vi "mod_Integer Rate Interpolation.vi"(4 "flush buffers? (F)":bool, 6 "reset? (T)":bool=TRUE, 9 "interpolation factor":i32=10, 11 "input[]":cdb[](array[numeric])) -> (3 "output[]":cdb[](array[numeric]), 5 "filter coefficients out[]":dbl[](array[numeric]))   [LabVIEW 2020, in "niAMT.lvlib"]
uses:
  <vilib>/addons/Modulation/niAMT.lvlib
  <vilib>/addons/Modulation/Analog/controls/mod_Integer Interpolator State.ctl
  nilvamt.dll
panel:
  in  "default state":T1
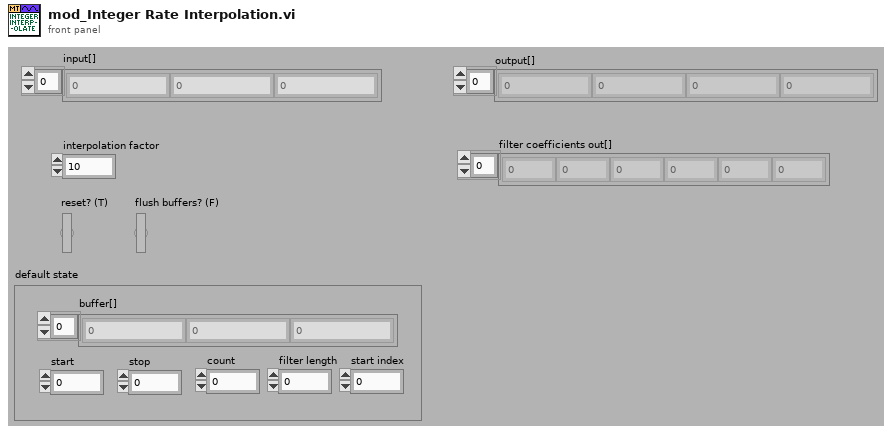
[diagram p1: front panel]
types:
  T1 = typedef "niAMT.lvlib/mod_Integer Interpolator State.ctl" = cluster{"buffer[]":cdb[], "start":i32, "stop":i32, "count":i32, "filter length":i32, "start index":i32}
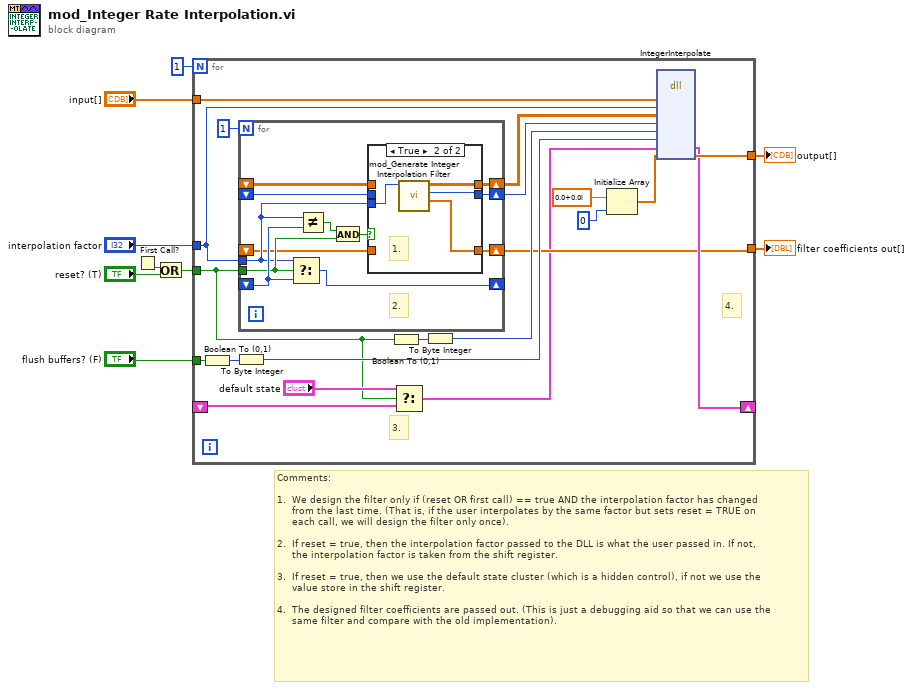
[diagram p0: block diagram]
diagram:
  # "Comments:\n\n1.  We design the filter only if (reset OR first call) == true AND the interpolation factor has changed\n     from the last time. (That is, if the user interpolates by the same factor but sets reset = TRUE on\n     each call, we will design the filter only once).\n\n2.  If reset = true, then the interpolation factor passed to the DLL is what the user passed in. If not,\n     the interpolation factor is taken from the shift register.\n\n3.  If reset = true, then we use the default state cluster (which is a hidden control), if not we use the\n     value store in the shift register.\n\n4.  The designed filter coefficients are passed out. (This is just a debugging aid so that we can use the\n     same filter and compare with the old implementation)."
  n1 = First Call?() -> (First Call?: T/F=w7:bool)
  n2 = Or(x=w7, y="reset? (T)") -> (x .or. y?=w6:bool)
  n3 = for {
    N: 1 -> [_]
    tunnel: "interpolation factor" -> [w26]
    tunnel: w6 -> [w10]
    shift-right: [w15] -> _
    shift-left: _ -> [w11]
    tunnel: "input[]" -> [w28]
    tunnel: "flush buffers? (F)" -> [w21]
    tunnel: [w16] -> w2
    tunnel: [w14] -> w1
    # "4."
    # "3."
    n4 = Boolean To (0,1)(Boolean=w21) -> (0, 1=w22:i16)
    n5 = To Byte Integer(number=w22) -> (8bit integer=w20:i8)
    n6 = for {
      N: 1 -> [_]
      shift-right: [w41] -> _
      shift-left: _ -> [w39]
      tunnel: w10 -> [w37]
      tunnel: w26 -> [w33]
      shift-right: [w40] -> w27
      shift-left: _ -> [w36]
      shift-right: [w35] -> w25
      shift-left: _ -> [w34]
      shift-right: [w32] -> w14
      shift-left: _ -> [w31]
      # "2."
      n7 = Select(t=w33, s=w37, f=w39) -> (s? t:f=w41:i32)
      n8 = Not Equal?(x=w33, y=w39) -> (x != y?=w38:bool)
      n9 = And(x=w38, y=w37) -> (x .and. y?=w30:bool)
      n10 = case shown="True" w30 {
        tunnel: [w44 w48] -> w40
        tunnel: w36 -> [w44 _]
        tunnel: [w43 w47] -> w35
        tunnel: w34 -> [w43 _]
        tunnel: w33 -> [_ w46]
        tunnel: [w42 w45] -> w32
        tunnel: w31 -> [w42 _]
        frame False {
        }
        frame True {
          # "1."
          n11 = call <vilib>:"mod_Generate Integer Interpolation Filter.vi"("interpolation factor"=w46) -> ("filter coefficients out"=w45:dbl[], "total length"=w47:i32, "polyphase filter out (2D)"=w48:dbl[][])  [unwired: 8 out]
        }
      }
    }
    n12 = Boolean To (0,1)(Boolean=w10) -> (0, 1=w24:i16)
    n13 = Select(t="default state", s=w10, f=w11) -> (s? t:f=w13:T1)
    n14 = To Byte Integer(number=w24) -> (8bit integer=w23:i8)
    n15 = Initialize Array(cdb 0.0+0.0i ("element"), 0 ("dimension size")) -> (w17:cdb[])
    n16 = dll-call lib="nilvamt.*" fn="IntegerInterpolate"("input"=w28, "interpolationFactor"=w26, "filter"=w27, "filterLength"=w25, "reset"=w23, "flush"=w20, "state"=w13, "output"=w17) -> ("state"=w15:T1, "output"=w16:cdb[])  [unwired: 9 in, 3 out]
  }
  "output[]" <- w2
  "filter coefficients out[]" <- w1
